vi "arm_calc.vi"() -> ()   [LabVIEW 2016]
uses:
  <vilib>/express/express arith-compare/Formula/XNode/ExpressFormulaBlockNode.xnode
  Control 1.ctl
panel:
  out "Result":dbl
  in  "L":T1
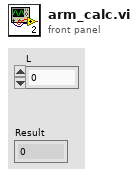
[diagram p1: front panel]
types:
  T1 = typedef "Control 1.ctl" = dbl
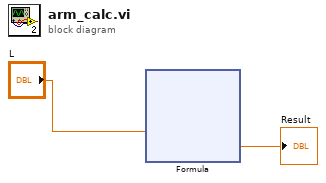
[diagram p0: block diagram]
diagram:
  n1 = xnode "Formula"("X1"="L") -> ("Result"=→"Result":dbl)  [unwired: 1 in, 1 out]
